vi "Read FIB Files.vi"() -> ()   [LabVIEW 2012]
panel:
  out "FIB parameters":T1
  out "SEM parameters":T2={"Detector A"="InLens", "Detector B"="Detector B", "Brightness A"=40.0, "Contrast A"=30.0, "Brightness B"=40.0, "Contrast B"=50.0, "Magnification"=5582.6, "Pixel size"=20.000582, "Working distance"=3.43328, "EHT"=1.1, "Aperture"=6, "High current mode"=1, "Probe current"=2.956808e-09, "Scan rotation"=0.0, "Chamber vac"=3.96371e-06, "Gun vac"=3.14396e-10, "Beam shift X"=0.0, "Beam shift Y"=0.0, "Stig X"=0.53615, "Stig Y"=-0.17615, "Alignment X"=-5.56036, "Alignment Y"=-13.20288, "Stage X"=52.5025, "Stage Y"=52.82977, "Stage Z"=18.42144, "Stage T"=54.0, "Stage R"=190.18593, "Stage M"=4.07375}
  out "Image Focus Index":T3={"A Img Focus Index"=0.26894957503947886, "B Img Focus Index"=11.996084418392877, "C Img Focus Index"=0.0, "D Img Focus Index"=0.0}
  in  "Image Tabs":T4(tab)
  out "Det D":sgl[][](graph)
  out "Det C":sgl[][](graph)
  out "Det B":sgl[][](graph)
  out "Det A":sgl[][](graph)
  out "Detector A":i16[][](graph) caption="InLens"
  out "Detector B":i16[][](graph) caption="ESB @ 600V"
  out "Detector C":i16[][](graph)
  out "Detector D":i16[][](graph)
  out "FIB shift X":sgl
  out "FIB shift Y":sgl
  out "FIB stig X":sgl
  out "FIB stig Y":sgl
  out "FIB align Y":sgl
  out "FIB align X":sgl
  out "FIB Rotation":sgl
  out "FIB current":sgl
  out "FIB probe":u8
  out "FIB focus":sgl
  out "Mode":u8
  out "Brightness B":sgl
  out "Contrast B":sgl
  out "Contrast A":sgl
  out "Brightness A":sgl
  out "Stage M":sgl
  out "Stage R":sgl
  out "Stage T":sgl
  out "Stage Z":sgl
  out "Stage Y":sgl
  out "Stage X":sgl
  out "SEM align X":sgl
  out "SEM align Y":sgl
  out "SEM stig X":sgl
  out "SEM stig Y":sgl
  out "SEM shift Y":sgl
  out "SEM shift X":sgl
  out "Gun vac":sgl
  out "Chamber vac":sgl
  out "SEM rotation":sgl
  out "SEM current":sgl
  out "High current":u8
  out "SEM Aperture":u8
  out "DetD":string
  out "DetC":string
  out "DetB":string
  out "DetA":string
  out "Notes":string
  out "EHT":sgl
  out "WD":sgl
  out "Pixel size":sgl
  out "Mag":sgl
  out "AI 4":bool
  out "AI 3":bool
  out "AI 2":bool
  out "AI 1":bool
  out "X max":sgl
  out "X min":sgl
  out "Frame line rampdown ratio":sgl
  out "Scan rate":sgl
  out "Zeiss scan speed":u8
  out "AI delay":i16
  out "Oversampling":u8
  out "Y resolution":u32
  out "X resolution":u32
  out "Scaling":sgl[][](array[numeric])
  out "Channel number":u8
  out "Time step":dbl
  out "File type":u16
  out "Vresion number":u16
  out "File length":dbl
  out "Magic number":u32
  out "error out":errorcluster
  in  "File path":path=path "E:/Images"
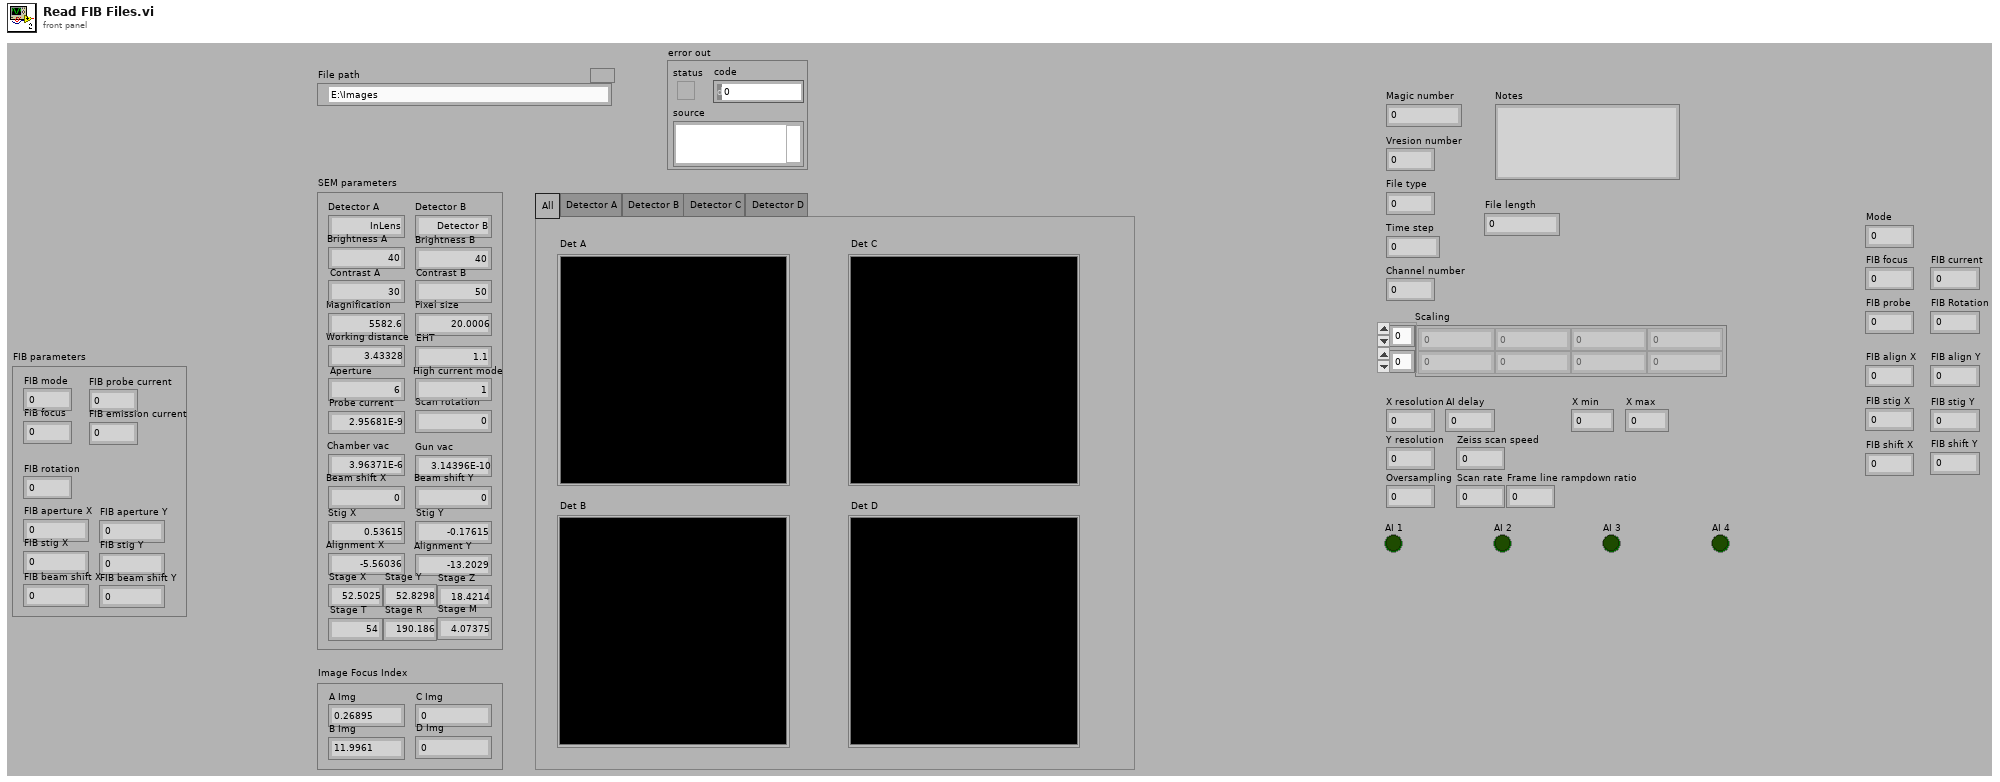
[diagram p1: front panel]
types:
  T1 = cluster{"FIB mode":u8, "FIB focus":sgl, "FIB probe current":u8, "FIB emission current":sgl, "FIB rotation":sgl, "FIB aperture X":sgl, "FIB aperture Y":sgl, "FIB stig X":sgl, "FIB stig Y":sgl, "FIB beam shift X":sgl, "FIB beam shift Y":sgl}
  T2 = cluster{"Detector A":string, "Detector B":string, "Brightness A":sgl, "Contrast A":sgl, "Brightness B":sgl, "Contrast B":sgl, "Magnification":sgl, "Pixel size":sgl, "Working distance":sgl, "EHT":sgl, "Aperture":u8, "High current mode":u8, "Probe current":sgl, "Scan rotation":sgl, "Chamber vac":sgl, "Gun vac":sgl, "Beam shift X":sgl, "Beam shift Y":sgl, "Stig X":sgl, "Stig Y":sgl, "Alignment X":sgl, "Alignment Y":sgl, "Stage X":sgl, "Stage Y":sgl, "Stage Z":sgl, "Stage T":sgl, "Stage R":sgl, "Stage M":sgl}
  T3 = cluster{"A Img Focus Index":dbl, "B Img Focus Index":dbl, "C Img Focus Index":dbl, "D Img Focus Index":dbl}
  T4 = enum32{"All", "Detector A", "Detector B", "Detector C", "Detector D"}
  T5 = enum16{"open", "replace", "create", "open or create", "replace or create", "replace or create with confirmation"}
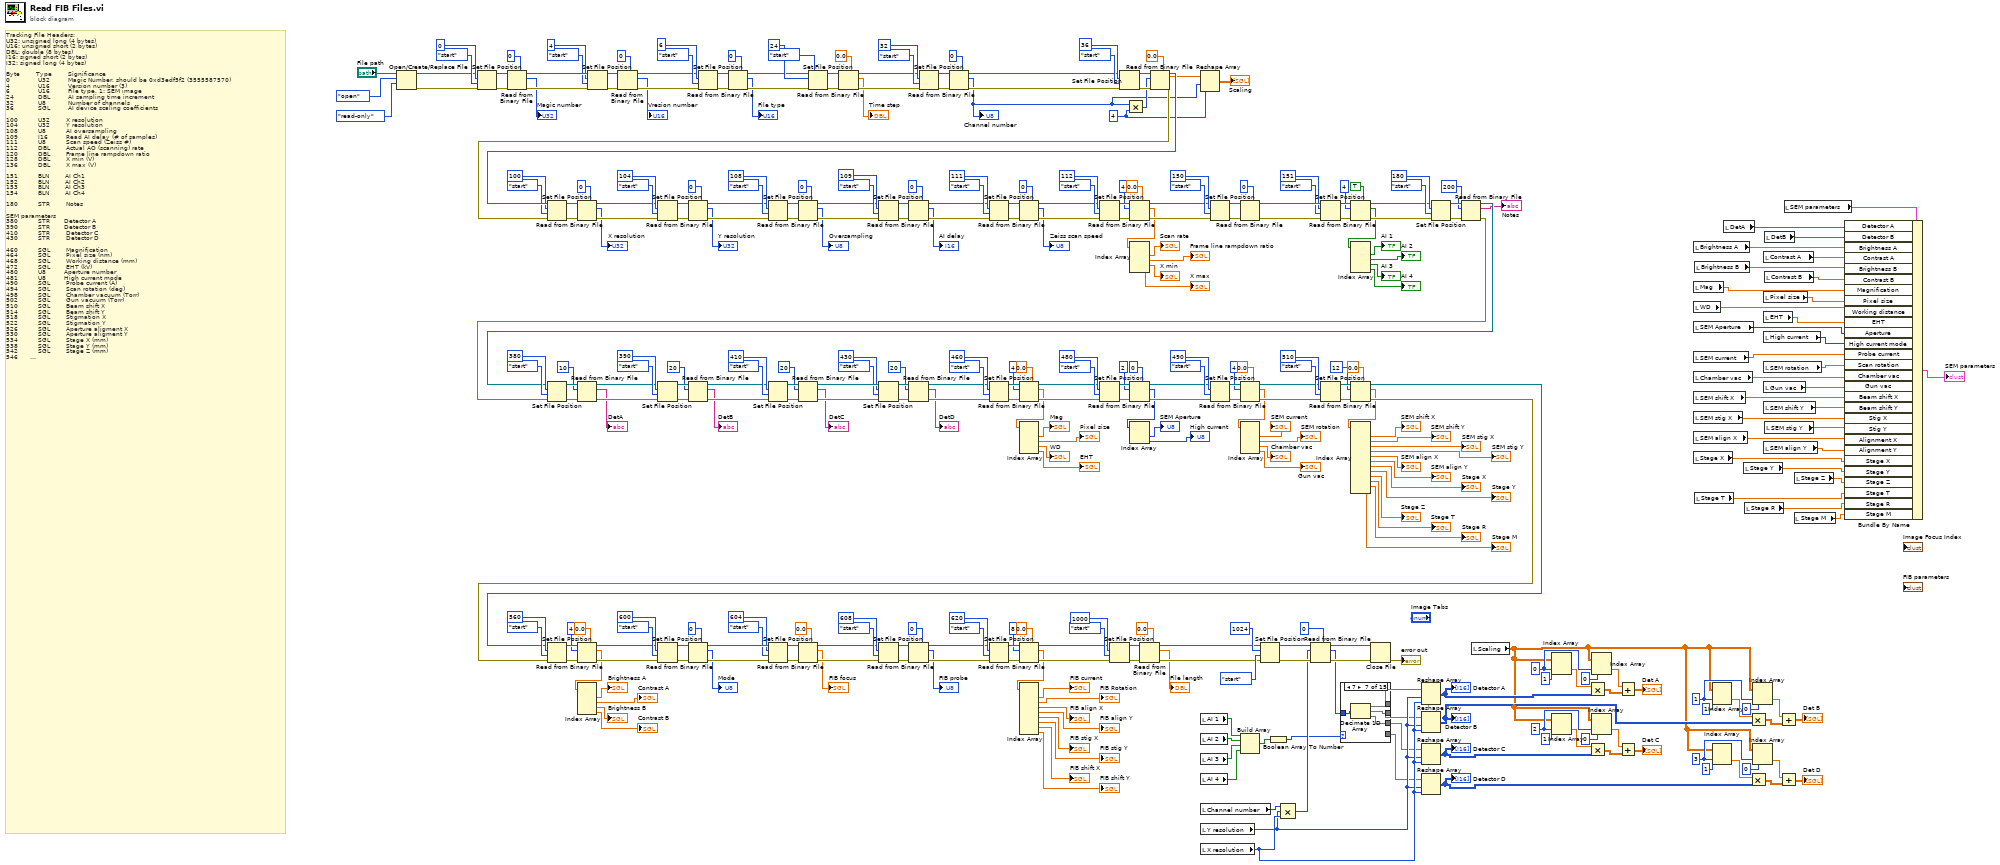
[diagram p0: block diagram]
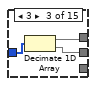
[diagram p4: hidden frame]
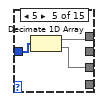
[diagram p6: hidden frame]
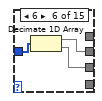
[diagram p7: hidden frame]
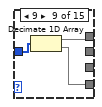
[diagram p9: hidden frame]
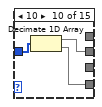
[diagram p10: hidden frame]
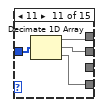
[diagram p11: hidden frame]
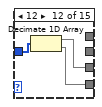
[diagram p12: hidden frame]
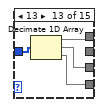
[diagram p13: hidden frame]
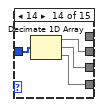
[diagram p14: hidden frame]
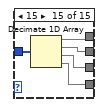
[diagram p15: hidden frame]
diagram:
  w47 = 3 ("index (row)")
  w37 = 2 ("index (row)")
  w48 = 1 ("index (row)")
  w62 = 0 ("index (row)")
  w148 = 4 ("count (1)")
  # "Tracking File Headers:\nU32: unsigned long (4 bytes)\nU16: unsigned short (2 bytes)\nDBL: double (8 bytes)\nI16: signed short (2 bytes)\nI32: signed long (4 bytes)\n\nByte\t       Type\t\t      Significance\n0              U32\t        Magic Number, should be 0xd3edf5f2 (3555587570)\n4   \t          U16\t        Version number (3)\n6   \t          U16\t        File type. 1: SEM image\n24     \t      DBL         AI sampling time increment\n32     \t      U8           Number of channels\n36            SGL         AI device scaling coefficients\n\n100          U32        X resolution\n104          U32        Y resolution\n108          U8          AI oversampling\n109          I16         Read AI delay (# of samples)\n111          U8          Scan speed (Zeiss #)\n112          DBL        Actual AO (scanning) rate\n120          DBL        Frame line rampdown ratio\n128          DBL        X min (V)\n136          DBL        X max (V)\n\n151          BLN        AI Ch1          \n152          BLN        AI Ch2\n153          BLN        AI Ch3\n154          BLN        AI Ch4\n \n180          STR        Notes\n\nSEM parameters\n380          STR       Detector A\n390          STR       Detector B\n410          STR        Detector C\n430          STR        Detector D\n\n460          SGL        Magnification\n464          SGL        Pixel size (nm)\n468          SGL        Working distance (mm)\n472          SGL        EHT (kV)\n480          U8         Aperture number\n481          U8         High current mode\n490          SGL        Probe current (A)\n494          SGL        Scan rotation (deg)\n498          SGL        Chamber vacuum (Torr)\n502          SGL        Gun vacuum (Torr)\n510          SGL        Beam shift X\n514          SGL        Beam shift Y\n518          SGL        Stigmation X\n522          SGL        Stigmation Y\n526          SGL        Aperture aligment X\n530          SGL        Aperture aligment Y\n534          SGL        Stage X (mm)\n538          SGL        Stage Y (mm)\n542          SGL        Stage Z (mm)\n546          SGL        Stage T (deg)\n550          SGL        Stage R (deg)\n554          SGL        Stage M (mm)\n560          SGL        Brightness (%), detector A\n564          SGL        Contrast (%),  detector A\n568          SGL        Brightness (%), detector B\n572          SGL        Contrast (%),  detector B\n\n\nFIB parameters\n600          U8         Mode\n604          SGL        Focus (V)\n608          U8         Probe current number\n620          SGL        Emission current (A)\n624          SGL        rotation (deg)\n628          SGL        Aperture alignment X\n632          SGL        Aperture alignment Y\n636          SGL        Stigmation X\n640          SGL        Stigmation Y\n644          SGL        Beam shift X (um)\n648          SGL        Beam shift Y (um)\n\n\n1000        DBL         File length\n\n1024        I16          1-D array of n channels of unscaled measurement from DAQ"
  n1 = Open/Create/Replace File(file path (use dialog)="File path", operation (0:open)=T5."open", access (0:read/write)=enum16{"read/write", "read-only", "write-only"}."read-only") -> (refnum out=w222:refnum<file>, error out=w221:errorcluster)  [unwired: 3 in, 1 out]
  n2 = Set File Position(offset (in bytes) (0)=0 ("pos offset (0)"), refnum=w222, from (0:start)=enum16{"start", "end", "current"}."start" ("pos mode (0:2)"), error in=w221) -> (refnum out=w332:refnum<file>, error out=w331:errorcluster)
  n3 = Read from Binary File(5:u32 0, 8:w331, 11:w332) -> (0:w361:errorcluster, 2:→"Magic number":u32, 3:w364:refnum<file>)  [unwired: 3 in, 1 out]
  n4 = Set File Position(offset (in bytes) (0)=4 ("pos offset (0)"), refnum=w364, from (0:start)=enum16{"start", "end", "current"}."start" ("pos mode (0:2)"), error in=w361) -> (refnum out=w334:refnum<file>, error out=w333:errorcluster)
  n5 = Read from Binary File(5:u16 0, 8:w333, 11:w334) -> (0:w357:errorcluster, 2:→"Vresion number":u16, 3:w358:refnum<file>)  [unwired: 3 in, 1 out]
  n6 = Set File Position(offset (in bytes) (0)=6 ("pos offset (0)"), refnum=w358, from (0:start)=enum16{"start", "end", "current"}."start" ("pos mode (0:2)"), error in=w357) -> (refnum out=w336:refnum<file>, error out=w335:errorcluster)
  n7 = Read from Binary File(5:u16 0, 8:w335, 11:w336) -> (0:w353:errorcluster, 2:→"File type":u16, 3:w354:refnum<file>)  [unwired: 3 in, 1 out]
  n8 = Set File Position(offset (in bytes) (0)=24 ("pos offset (0)"), refnum=w354, from (0:start)=enum16{"start", "end", "current"}."start" ("pos mode (0:2)"), error in=w353) -> (refnum out=w338:refnum<file>, error out=w337:errorcluster)
  n9 = Read from Binary File(5:0.0 ("1/x"), 8:w337, 11:w338) -> (0:w349:errorcluster, 2:→"Time step":dbl, 3:w350:refnum<file>)  [unwired: 3 in, 1 out]
  n10 = Set File Position(offset (in bytes) (0)=32 ("pos offset (0)"), refnum=w350, from (0:start)=enum16{"start", "end", "current"}."start" ("pos mode (0:2)"), error in=w349) -> (refnum out=w340:refnum<file>, error out=w339:errorcluster)
  n11 = Read from Binary File(5:u8 0 ("unsigned 8bit integer"), 8:w339, 11:w340) -> (0:w345:errorcluster, 2:w149:u8, 3:w346:refnum<file>)  [unwired: 3 in, 1 out]
  "Channel number" <- w149
  n12 = Set File Position(offset (in bytes) (0)=36 ("pos offset (0)"), refnum=w346, from (0:start)=enum16{"start", "end", "current"}."start" ("pos mode (0:2)"), error in=w345) -> (refnum out=w342:refnum<file>, error out=w341:errorcluster)
  n13 = Multiply(x=w149, y=w148) -> (x*y=w151:i32)
  n14 = Read from Binary File(5:sgl 0.0, 8:w341, 10:w151, 11:w342) -> (0:w329:errorcluster, 2:w150:sgl[], 3:w330:refnum<file>)  [unwired: 2 in, 1 out]
  n15 = Set File Position(offset (in bytes) (0)=100 ("pos offset (0)"), refnum=w330, from (0:start)=enum16{"start", "end", "current"}."start" ("pos mode (0:2)"), error in=w329) -> (refnum out=w323:refnum<file>, error out=w324:errorcluster)
  n16 = Read from Binary File(5:u32 0 ("X resolution"), 8:w324, 11:w323) -> (0:w303:errorcluster, 2:→"X resolution":u32, 3:w304:refnum<file>)  [unwired: 3 in, 1 out]
  n17 = Set File Position(offset (in bytes) (0)=104 ("pos offset (0)"), refnum=w304, from (0:start)=enum16{"start", "end", "current"}."start" ("pos mode (0:2)"), error in=w303) -> (refnum out=w318:refnum<file>, error out=w317:errorcluster)
  n18 = Read from Binary File(5:u32 0 ("Y resolution"), 8:w317, 11:w318) -> (0:w305:errorcluster, 2:→"Y resolution":u32, 3:w306:refnum<file>)  [unwired: 3 in, 1 out]
  n19 = Set File Position(offset (in bytes) (0)=108 ("pos offset (0)"), refnum=w306, from (0:start)=enum16{"start", "end", "current"}."start" ("pos mode (0:2)"), error in=w305) -> (refnum out=w315:refnum<file>, error out=w316:errorcluster)
  n20 = Read from Binary File(5:u8 0 ("unsigned 8bit integer"), 8:w316, 11:w315) -> (0:w307:errorcluster, 2:→"Oversampling":u8, 3:w308:refnum<file>)  [unwired: 3 in, 1 out]
  n21 = Set File Position(offset (in bytes) (0)=109 ("pos offset (0)"), refnum=w308, from (0:start)=enum16{"start", "end", "current"}."start" ("pos mode (0:2)"), error in=w307) -> (refnum out=w310:refnum<file>, error out=w309:errorcluster)
  n22 = Read from Binary File(5:i16 0 ("Read AI delay"), 8:w309, 11:w310) -> (0:w297:errorcluster, 2:→"AI delay":i16, 3:w298:refnum<file>)  [unwired: 3 in, 1 out]
  n23 = Set File Position(offset (in bytes) (0)=111 ("pos offset (0)"), refnum=w298, from (0:start)=enum16{"start", "end", "current"}."start" ("pos mode (0:2)"), error in=w297) -> (refnum out=w300:refnum<file>, error out=w299:errorcluster)
  n24 = Read from Binary File(5:u8 0 ("Scan speed"), 8:w299, 11:w300) -> (0:w291:errorcluster, 2:→"Zeiss scan speed":u8, 3:w292:refnum<file>)  [unwired: 3 in, 1 out]
  n25 = Set File Position(offset (in bytes) (0)=112 ("pos offset (0)"), refnum=w292, from (0:start)=enum16{"start", "end", "current"}."start" ("pos mode (0:2)"), error in=w291) -> (refnum out=w295:refnum<file>, error out=w296:errorcluster)
  n26 = Read from Binary File(5:0.0, 8:w296, 10:4 ("count (1)"), 11:w295) -> (0:w285:errorcluster, 2:w141:dbl[], 3:w286:refnum<file>)  [unwired: 2 in, 1 out]
  n27 = Index Array(array=w141) -> (element #1=→"Scan rate":dbl, element #2=→"Frame line rampdown ratio":dbl, element #3=→"X min":dbl, element #4=→"X max":dbl)  [unwired: 4 in]
  n28 = Reshape Array(w150, w149, w148) -> (→"Scaling":sgl[][])
  n29 = local read "AI 1"() -> (w73:bool)
  n30 = local read "AI 2"() -> (w72:bool)
  n31 = local read "AI 3"() -> (w71:bool)
  n32 = local read "AI 4"() -> (w70:bool)
  n33 = local read "Channel number"() -> (w77:u8)
  n34 = local read "Y resolution"() -> (w68:u32)
  n35 = local read "X resolution"() -> (w69:u32)
  n36 = Set File Position(offset (in bytes) (0)=150 ("pos offset (0)"), refnum=w286, from (0:start)=enum16{"start", "end", "current"}."start" ("pos mode (0:2)"), error in=w285) -> (refnum out=w289:refnum<file>, error out=w290:errorcluster)
  n37 = Read from Binary File(5:0 ("pos offset (0)"), 8:w290, 11:w289) -> (0:w283:errorcluster, 3:w284:refnum<file>)  [unwired: 3 in, 2 out]
  n38 = Build Array(w73, w72, w71, w70) -> (w76:bool[])
  n39 = Boolean Array To Number(Boolean array=w76) -> (number=w75:u32)
  n40 = Compound Arithmetic op=MULTIPLY(w77, w68, w69) -> (w78:u32)
  n41 = Set File Position(offset (in bytes) (0)=151 ("pos offset (0)"), refnum=w284, from (0:start)=enum16{"start", "end", "current"}."start" ("pos mode (0:2)"), error in=w283) -> (refnum out=w276:refnum<file>, error out=w275:errorcluster)
  n42 = Read from Binary File(5:TRUE ("AI 4"), 8:w275, 10:4 ("count (1)"), 11:w276) -> (0:w225:errorcluster, 2:w136:bool[], 3:w226:refnum<file>)  [unwired: 2 in, 1 out]
  n43 = Index Array(array=w136) -> (element #1=→"AI 1":bool, element #2=→"AI 2":bool, element #3=→"AI 3":bool, element #4=→"AI 4":bool)  [unwired: 4 in]
  n44 = Set File Position(offset (in bytes) (0)=180 ("pos offset (0)"), refnum=w226, from (0:start)=enum16{"start", "end", "current"}."start" ("pos mode (0:2)"), error in=w225) -> (refnum out=w280:refnum<file>, error out=w279:errorcluster)
  n45 = Read from Binary File(8:w279, 10:200 ("count (1)"), 11:w280) -> (0:w227:errorcluster, 2:→"Notes":string, 3:w228:refnum<file>)  [unwired: 3 in, 1 out]
  n46 = Set File Position(offset (in bytes) (0)=380 ("pos offset (0)"), refnum=w228, from (0:start)=enum16{"start", "end", "current"}."start" ("pos mode (0:2)"), error in=w227) -> (refnum out=w256:refnum<file>, error out=w255:errorcluster)
  n47 = Read from Binary File(8:w255, 10:10 ("count (1)"), 11:w256) -> (0:w245:errorcluster, 2:→"DetA":string, 3:w246:refnum<file>)  [unwired: 3 in, 1 out]
  n48 = Set File Position(offset (in bytes) (0)=390 ("pos offset (0)"), refnum=w246, from (0:start)=enum16{"start", "end", "current"}."start" ("pos mode (0:2)"), error in=w245) -> (refnum out=w248:refnum<file>, error out=w247:errorcluster)
  n49 = Read from Binary File(8:w247, 10:20 ("count (1)"), 11:w248) -> (0:w233:errorcluster, 2:→"DetB":string, 3:w234:refnum<file>)  [unwired: 3 in, 1 out]
  n50 = Set File Position(offset (in bytes) (0)=410 ("pos offset (0)"), refnum=w234, from (0:start)=enum16{"start", "end", "current"}."start" ("pos mode (0:2)"), error in=w233) -> (refnum out=w241:refnum<file>, error out=w242:errorcluster)
  n51 = Read from Binary File(8:w242, 10:20 ("count (1)"), 11:w241) -> (0:w244:errorcluster, 2:→"DetC":string, 3:w243:refnum<file>)  [unwired: 3 in, 1 out]
  n52 = Set File Position(offset (in bytes) (0)=430 ("pos offset (0)"), refnum=w243, from (0:start)=enum16{"start", "end", "current"}."start" ("pos mode (0:2)"), error in=w244) -> (refnum out=w236:refnum<file>, error out=w235:errorcluster)
  n53 = Read from Binary File(8:w235, 10:20 ("count (1)"), 11:w236) -> (0:w231:errorcluster, 2:→"DetD":string, 3:w232:refnum<file>)  [unwired: 3 in, 1 out]
  n54 = Set File Position(offset (in bytes) (0)=460 ("pos offset (0)"), refnum=w232, from (0:start)=enum16{"start", "end", "current"}."start" ("pos mode (0:2)"), error in=w231) -> (refnum out=w258:refnum<file>, error out=w257:errorcluster)
  n55 = Read from Binary File(5:sgl 0.0 ("EHT"), 8:w257, 10:4 ("count (1)"), 11:w258) -> (0:w267:errorcluster, 2:w128:sgl[], 3:w268:refnum<file>)  [unwired: 2 in, 1 out]
  n56 = Index Array(array=w128) -> (element #1=→"Mag":sgl, element #2=→"Pixel size":sgl, element #3=→"WD":sgl, element #4=→"EHT":sgl)  [unwired: 4 in]
  n57 = Set File Position(offset (in bytes) (0)=480 ("pos offset (0)"), refnum=w268, from (0:start)=enum16{"start", "end", "current"}."start" ("pos mode (0:2)"), error in=w267) -> (refnum out=w260:refnum<file>, error out=w259:errorcluster)
  n58 = Read from Binary File(5:u8 0 ("High current mode"), 8:w259, 10:2 ("count (1)"), 11:w260) -> (0:w263:errorcluster, 2:w116:u8[], 3:w264:refnum<file>)  [unwired: 2 in, 1 out]
  n59 = Index Array(array=w116) -> (element #1=→"SEM Aperture":u8, element #2=→"High current":u8)  [unwired: 2 in]
  n60 = Set File Position(offset (in bytes) (0)=490 ("pos offset (0)"), refnum=w264, from (0:start)=enum16{"start", "end", "current"}."start" ("pos mode (0:2)"), error in=w263) -> (refnum out=w262:refnum<file>, error out=w261:errorcluster)
  n61 = Read from Binary File(5:sgl 0.0 ("Gun vac"), 8:w261, 10:4 ("count (1)"), 11:w262) -> (0:w223:errorcluster, 2:w113:sgl[], 3:w224:refnum<file>)  [unwired: 2 in, 1 out]
  n62 = Index Array(array=w113) -> (element #1=→"SEM current":sgl, element #2=→"SEM rotation":sgl, element #3=→"Chamber vac":sgl, element #4=→"Gun vac":sgl)  [unwired: 4 in]
  n63 = Set File Position(offset (in bytes) (0)=510 ("pos offset (0)"), refnum=w224, from (0:start)=enum16{"start", "end", "current"}."start" ("pos mode (0:2)"), error in=w223) -> (refnum out=w253:refnum<file>, error out=w254:errorcluster)
  n64 = Read from Binary File(5:sgl 0.0 ("Stage M"), 8:w254, 10:12 ("count (1)"), 11:w253) -> (0:w229:errorcluster, 2:w108:sgl[], 3:w230:refnum<file>)  [unwired: 2 in, 1 out]
  n65 = Set File Position(offset (in bytes) (0)=560 ("pos offset (0)"), refnum=w230, from (0:start)=enum16{"start", "end", "current"}."start" ("pos mode (0:2)"), error in=w229) -> (refnum out=w327:refnum<file>, error out=w328:errorcluster)
  n66 = Read from Binary File(5:sgl 0.0 ("Contrast B"), 8:w328, 10:4 ("count (1)"), 11:w327) -> (0:w158:errorcluster, 2:w95:sgl[], 3:w157:refnum<file>)  [unwired: 2 in, 1 out]
  n67 = Index Array(array=w95) -> (element #1=→"Brightness A":sgl, element #2=→"Contrast A":sgl, element #3=→"Brightness B":sgl, element #4=→"Contrast B":sgl)  [unwired: 4 in]
  n68 = Set File Position(offset (in bytes) (0)=600 ("pos offset (0)"), refnum=w157, from (0:start)=enum16{"start", "end", "current"}."start" ("pos mode (0:2)"), error in=w158) -> (refnum out=w193:refnum<file>, error out=w194:errorcluster)
  n69 = Read from Binary File(5:u8 0 ("FIB mode"), 8:w194, 11:w193) -> (0:w189:errorcluster, 2:→"Mode":u8, 3:w190:refnum<file>)  [unwired: 3 in, 1 out]
  n70 = Set File Position(offset (in bytes) (0)=604 ("pos offset (0)"), refnum=w190, from (0:start)=enum16{"start", "end", "current"}."start" ("pos mode (0:2)"), error in=w189) -> (refnum out=w174:refnum<file>, error out=w173:errorcluster)
  n71 = Read from Binary File(5:sgl 0.0 ("FIB focus"), 8:w173, 11:w174) -> (0:w183:errorcluster, 2:→"FIB focus":sgl, 3:w184:refnum<file>)  [unwired: 3 in, 1 out]
  n72 = Set File Position(offset (in bytes) (0)=608 ("pos offset (0)"), refnum=w184, from (0:start)=enum16{"start", "end", "current"}."start" ("pos mode (0:2)"), error in=w183) -> (refnum out=w176:refnum<file>, error out=w175:errorcluster)
  n73 = Read from Binary File(5:u8 0 ("FIB probe current"), 8:w175, 11:w176) -> (0:w179:errorcluster, 2:→"FIB probe":u8, 3:w180:refnum<file>)  [unwired: 3 in, 1 out]
  n74 = Set File Position(offset (in bytes) (0)=620 ("pos offset (0)"), refnum=w180, from (0:start)=enum16{"start", "end", "current"}."start" ("pos mode (0:2)"), error in=w179) -> (refnum out=w178:refnum<file>, error out=w177:errorcluster)
  n75 = Read from Binary File(5:sgl 0.0 ("FIB focus"), 8:w177, 10:8 ("count (1)"), 11:w178) -> (0:w159:errorcluster, 2:w87:sgl[], 3:w160:refnum<file>)  [unwired: 2 in, 1 out]
  n76 = Index Array(array=w87) -> (element #1=→"FIB current":sgl, element #2=→"FIB Rotation":sgl, element #3=→"FIB align X":sgl, element #4=→"FIB align Y":sgl, element #5=→"FIB stig X":sgl, element #6=→"FIB stig Y":sgl, element #7=→"FIB shift X":sgl, element #8=→"FIB shift Y":sgl)  [unwired: 8 in]
  n77 = Set File Position(offset (in bytes) (0)=1000 ("pos offset (0)"), refnum=w160, from (0:start)=enum16{"start", "end", "current"}."start" ("pos mode (0:2)"), error in=w159) -> (refnum out=w165:refnum<file>, error out=w166:errorcluster)
  n78 = Read from Binary File(5:0.0 ("FIB focus"), 8:w166, 11:w165) -> (0:w161:errorcluster, 2:→"File length":dbl, 3:w162:refnum<file>)  [unwired: 3 in, 1 out]
  n79 = Set File Position(offset (in bytes) (0)=i64 1024, refnum=w162, from (0:start)=enum16{"start", "end", "current"}."start", error in=w161) -> (refnum out=w369:refnum<file>, error out=w368:errorcluster)
  n80 = Read from Binary File(5:i16 0, 8:w368, 10:w78, 11:w369) -> (0:w371:errorcluster, 2:w74:i16[], 3:w372:refnum<file>)  [unwired: 2 in, 1 out]
  n81 = case shown="7" w75 {
    tunnel: [w376 _ w380 _ w383 _ w390 _ w394 _ w401 _ w408 _ w417] -> w67
    tunnel: w74 -> [w376 w377 w379 w381 w384 w385 w391 w392 w395 w398 w402 w405 w409 w413 w418]
    tunnel: [_ w377 w378 _ _ w387 w389 _ _ w397 w400 _ _ w412 w416] -> w66
    tunnel: [_ _ _ w381 w382 w386 w388 _ _ _ _ w404 w407 w410 w415] -> w65
    tunnel: [_ _ _ _ _ _ _ w392 w393 w396 w399 w403 w406 w411 w414] -> w64
    frame 1, Default {
    }
    frame 2 {
    }
    frame 3 {
      n82 = Decimate 1D Array(w379) -> (w380:i16[], w378:i16[])
    }
    frame 4 {
    }
    frame 5 {
      n83 = Decimate 1D Array(w384) -> (w383:i16[], w382:i16[])
    }
    frame 6 {
      n84 = Decimate 1D Array(w385) -> (w387:i16[], w386:i16[])
    }
    frame 7 {
      n85 = Decimate 1D Array(w391) -> (w390:i16[], w389:i16[], w388:i16[])
    }
    frame 8 {
    }
    frame 9 {
      n86 = Decimate 1D Array(w395) -> (w394:i16[], w393:i16[])
    }
    frame 10 {
      n87 = Decimate 1D Array(w398) -> (w397:i16[], w396:i16[])
    }
    frame 11 {
      n88 = Decimate 1D Array(w402) -> (w401:i16[], w400:i16[], w399:i16[])
    }
    frame 12 {
      n89 = Decimate 1D Array(w405) -> (w404:i16[], w403:i16[])
    }
    frame 13 {
      n90 = Decimate 1D Array(w409) -> (w408:i16[], w407:i16[], w406:i16[])
    }
    frame 14 {
      n91 = Decimate 1D Array(w413) -> (w412:i16[], w410:i16[], w411:i16[])
    }
    frame 15 {
      n92 = Decimate 1D Array(w418) -> (w417:i16[], w416:i16[], w415:i16[], w414:i16[])
    }
  }
  n93 = Index Array(array=w108) -> (element #1=→"SEM shift X":sgl, element #2=→"SEM shift Y":sgl, element #3=→"SEM stig X":sgl, element #4=→"SEM stig Y":sgl, element #5=→"SEM align X":sgl, element #6=→"SEM align Y":sgl, element #7=→"Stage X":sgl, element #8=→"Stage Y":sgl, element #9=→"Stage Z":sgl, element #10=→"Stage T":sgl, element #11=→"Stage R":sgl, element #12=→"Stage M":sgl)  [unwired: 12 in]
  n94 = Close File(refnum=w372, error in=w371) -> (error out=→"error out":errorcluster)  [unwired: 1 out]
  n95 = Reshape Array(w67, w68, w69) -> (w57:i16[][])
  "Detector A" <- w57
  n96 = Reshape Array(w66, w68, w69) -> (w49:i16[][])
  "Detector B" <- w49
  n97 = Reshape Array(w65, w68, w69) -> (w34:i16[][])
  "Detector C" <- w34
  n98 = Reshape Array(w64, w68, w69) -> (w31:i16[][])
  "Detector D" <- w31
  n99 = local read "Scaling"() -> (w35:sgl[][])
  n100 = Index Array(array=w35, index (row)=w62, index (col)=1) -> (element=w59:sgl)
  n101 = Index Array(array=w35, index (row)=w37, index (col)=1) -> (element=w40:sgl)
  n102 = Multiply(x=w59, y=w57) -> (x*y=w58:sgl[][])
  n103 = Multiply(x=w40, y=w34) -> (x*y=w41:sgl[][])
  n104 = Index Array(array=w35, index (row)=w62, index (col)=0 ("disabled index (col)")) -> (element=w60:sgl)
  n105 = Index Array(array=w35, index (row)=w37, index (col)=0 ("disabled index (col)")) -> (element=w39:sgl)
  n106 = Add(x=w60, y=w58) -> (x+y=→"Det A":sgl[][])
  n107 = Add(x=w39, y=w41) -> (x+y=→"Det C":sgl[][])
  n108 = local read "Brightness A"() -> (w26:sgl)
  n109 = local read "Mag"() -> (w22:sgl)
  n110 = local read "WD"() -> (w20:sgl)
  n111 = local read "SEM Aperture"() -> (w17:u8)
  n112 = local read "SEM current"() -> (w13:sgl)
  n113 = local read "Chamber vac"() -> (w15:sgl)
  n114 = local read "SEM shift X"() -> (w7:sgl)
  n115 = local read "SEM stig X"() -> (w9:sgl)
  n116 = local read "SEM align X"() -> (w11:sgl)
  n117 = local read "Stage X"() -> (w1:sgl)
  n118 = local read "Brightness B"() -> (w23:sgl)
  n119 = local read "Stage T"() -> (w4:sgl)
  n120 = Index Array(array=w35, index (row)=w48, index (col)=1) -> (element=w52:sgl)
  n121 = Index Array(array=w35, index (row)=w47, index (col)=1) -> (element=w45:sgl)
  n122 = local read "DetA"() -> (w28:string)
  n123 = local read "Stage Y"() -> (w2:sgl)
  n124 = local read "Stage R"() -> (w5:sgl)
  n125 = Multiply(x=w52, y=w49) -> (x*y=w53:sgl[][])
  n126 = Multiply(x=w45, y=w31) -> (x*y=w44:sgl[][])
  n127 = Index Array(array=w35, index (row)=w48, index (col)=0 ("disabled index (col)")) -> (element=w51:sgl)
  n128 = Index Array(array=w35, index (row)=w47, index (col)=0 ("disabled index (col)")) -> (element=w46:sgl)
  n129 = local read "Contrast A"() -> (w25:sgl)
  n130 = local read "Pixel size"() -> (w21:sgl)
  n131 = local read "EHT"() -> (w19:sgl)
  n132 = local read "High current"() -> (w18:u8)
  n133 = local read "SEM rotation"() -> (w14:sgl)
  n134 = local read "Gun vac"() -> (w16:sgl)
  n135 = local read "SEM shift Y"() -> (w8:sgl)
  n136 = local read "SEM align Y"() -> (w12:sgl)
  n137 = local read "DetB"() -> (w27:string)
  n138 = local read "Contrast B"() -> (w24:sgl)
  n139 = local read "SEM stig Y"() -> (w10:sgl)
  n140 = Add(x=w51, y=w53) -> (x+y=→"Det B":sgl[][])
  n141 = Add(x=w46, y=w44) -> (x+y=→"Det D":sgl[][])
  n142 = local read "SEM parameters"() -> (w30:T2)
  n143 = local read "Stage M"() -> (w6:sgl)
  n144 = local read "Stage Z"() -> (w3:sgl)
  n145 = Bundle By Name(cluster=w30, "Detector A"=w28, "Detector B"=w27, "Brightness A"=w26, "Contrast A"=w25, "Brightness B"=w23, "Contrast B"=w24, "Magnification"=w22, "Pixel size"=w21, "Working distance"=w20, "EHT"=w19, "Aperture"=w17, "High current mode"=w18, "Probe current"=w13, "Scan rotation"=w14, "Chamber vac"=w15, "Gun vac"=w16, "Beam shift X"=w7, "Beam shift Y"=w8, "Stig X"=w9, "Stig Y"=w10, "Alignment X"=w11, "Alignment Y"=w12, "Stage X"=w1, "Stage Y"=w2, "Stage Z"=w3, "Stage T"=w4, "Stage R"=w5, "Stage M"=w6) -> (→"SEM parameters":T2)
